vi "FPGA - Revert (ECAT).vi"(8 "error in (no error)":errorcluster, 11 "Node Ptr":u64 format="%.0x") -> (0 "error out":errorcluster)   [LabVIEW 2019, in "SEECD System Explorer.lvlib"]
uses:
  SEECD System Explorer.lvlib
panel:
  in  "Tag":string
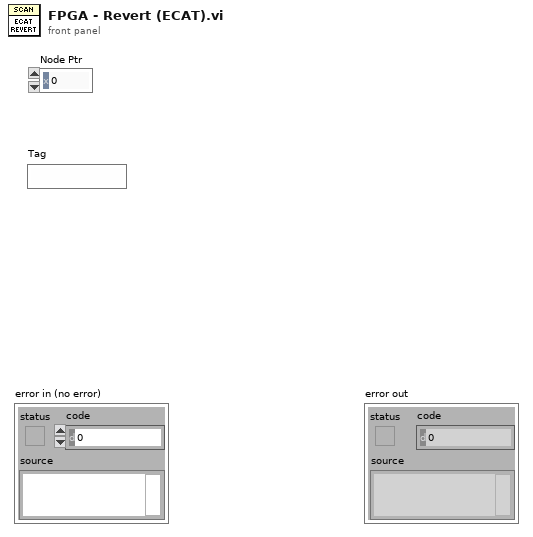
[diagram p1: front panel]
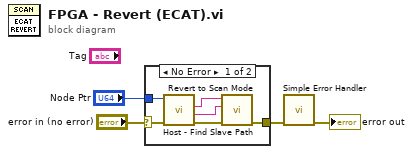
[diagram p0: block diagram]
diagram:
  n1 = case shown="No Error" "error in (no error)" {
    selector: "error in (no error)" -> [w7 w11]
    tunnel: "Node Ptr" -> [w5 _]
    tunnel: [w6 w11] -> w2
    frame No Error {
      n2 = call "Host - Find Slave Path.vi"("error in (no error)"=w7, "Item Ref in"=w5) -> ("error out"=w8:errorcluster, "Target IP Address"=w10:string, "Slave Ref"=w9:string)  [unwired: 6 in, 1 out]
      n3 = call "Revert to Scan Mode.vi"("error in"=w8, "Target IP Address"=w10, "Slave Ref"=w9) -> ("error out"=w6:errorcluster)  [unwired: 8 in]
    }
    frame Error {
    }
  }
  n4 = call <vilib>:"Simple Error Handler.vi"("error in (no error)"=w2) -> ("error out"=→"error out":errorcluster)  [unwired: 4 in, 4 out]
